vi "Swerve Wheel.vi"(7 "Wheel":T1(ring), 10 "Inputs":dbl[](array[numeric])) -> (1 "Speed":dbl, 2 "Motor Output":dbl)   [LabVIEW 2017]
uses:
  Public/Documents/Cross The Road Electronics/Phoenix-LabVIEW/Motor Controller/Controls/CTRE_Phoenix_MotorControl_ControlMode.ctl
  <vilib>/Rock Robotics/Network Tables/NT Read Number.vi
  <vilib>/Rock Robotics/Network Tables/NT Write Number.vi
  <vilib>/Rock Robotics/Network Tables/NT Read Numeric Array.vi
  <vilib>/addons/control/pid/pid.llb/PID (DBL).vi
  <vilib>/addons/control/pid/NI_PID_pid.lvlib
panel:
  out "PID Values":cluster{"P":dbl, "I":dbl, "D":dbl}
  # "Swerve Wheel Control\nFRC Team 34"
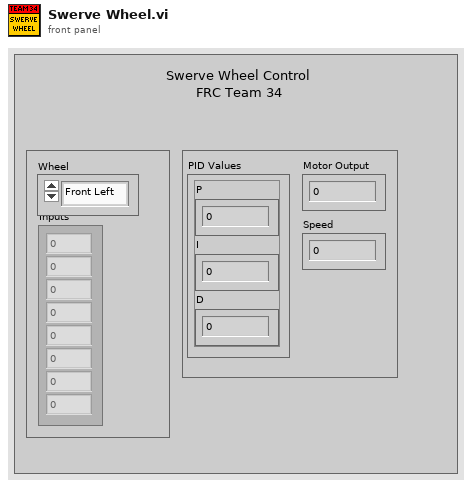
[diagram p1: front panel]
types:
  T1 = enum16{"Front Left", "Front Right", "Back Left", "Back Right"}
  T2 = typedef "CTRE_Phoenix_MotorControl_ControlMode.ctl" = u16
  T3 = enum16{"Z", "Y", "X", "Rot. Point X", "Rot. Point Y", "Width/2", "Max", "Length/2"}
  T4 = enum16{"Z Axis", "Y", "X", "Rot. Point X", "Rot. Point Y", "Width/2", "Max", "Length/2"}
  T5 = typedef "WPI_MotorControlDeviceRef.ctl" = cluster{"DeviceStatus":errorcluster, "Type":T6, "PWM":cluster{"PWM Channel":T7, "DeadBand":T8}, "CAN":cluster{"Device Number":u8, "SetOutput VI Ref":variant, "GetOutput VI Ref":variant, "Enable VI Ref":variant, "Disable VI Ref":variant, "Data":variant}, "Invert":bool, "DIO PWM":cluster{"PWM \"Enable\" Channel":T7, "DIOChannel":T9, "PWM Rate":dbl}}
  T6 = typedef "WPI_MotorControlType.ctl" = enum16{"PWM", "CAN", "DIO PWM"}
  T7 = typedef "FPGA_DIOPWMChannel.ctl" = enum8{"PWM 0", "PWM 1", "PWM 2", "PWM 3", "PWM 4", "PWM 5", "PWM 6", "PWM 7", "PWM 8", "PWM 9", "PWM MXP 0", "PWM MXP 1", "PWM MXP 2", "PWM MXP 3", "PWM MXP 4", "PWM MXP 5", "PWM MXP 6", "PWM MXP 7", "PWM MXP 8", "PWM MXP 9", "Invalid"}
  T8 = typedef "WPI_PWMDeadband.ctl" = cluster{"Name":string, "maxPositivePwm":i32, "minPositivePwm":i32, "centerPwm":i32, "maxNegativePwm":i32, "minNegativePwm":i32, "angularRange":u16}
  T9 = typedef "FPGA_DIOChannel.ctl" = enum8{"DIO 0", "DIO 1", "DIO 2", "DIO 3", "DIO 4", "DIO 5", "DIO 6", "DIO 7", "DIO 8", "DIO 9", "DIO MXP 0", "DIO MXP 1", "DIO MXP 2", "DIO MXP 3", "DIO MXP 4", "DIO MXP 5", "DIO MXP 6", "DIO MXP 7", "DIO MXP 8", "DIO MXP 9", "DIO MXP 10", "DIO MXP 11", "DIO MXP 12", "DIO MXP 13", "DIO MXP 14", "DIO MXP 15", "SPI Port CS1", "SPI Port CS2", "SPI Port CS3", "SPI Port MISO", "SPI Port MOSI", "Invalid"}
  T10 = typedef "WPI_EncoderDevRef.ctl" = cluster{"DevStatus":errorcluster, "EncoderIndex":T11, "CounterIndex":T12, "DistancePerCount":dbl, "Decoding Type":T13}
  T11 = typedef "FPGA_EncoderIdx.ctl" = enum8{"Enc 0", "Enc 1", "Enc 2", "Enc 3", "Enc 4", "Enc 5", "Enc 6", "Enc 7", "Invalid"}
  T12 = typedef "FPGA_CounterCtrSystemIndex.ctl" = enum8{"Ctr 0", "Ctr 1", "Ctr 2", "Ctr 3", "Ctr 4", "Ctr 5", "Ctr 6", "Ctr 7", "Invalid"}
  T13 = typedef "WPI_EncoderType.ctl" = enum16{"1x", "2x", "4x"}
  T14 = cluster{"Numeric":dbl, "Numeric":dbl, "Numeric":dbl}
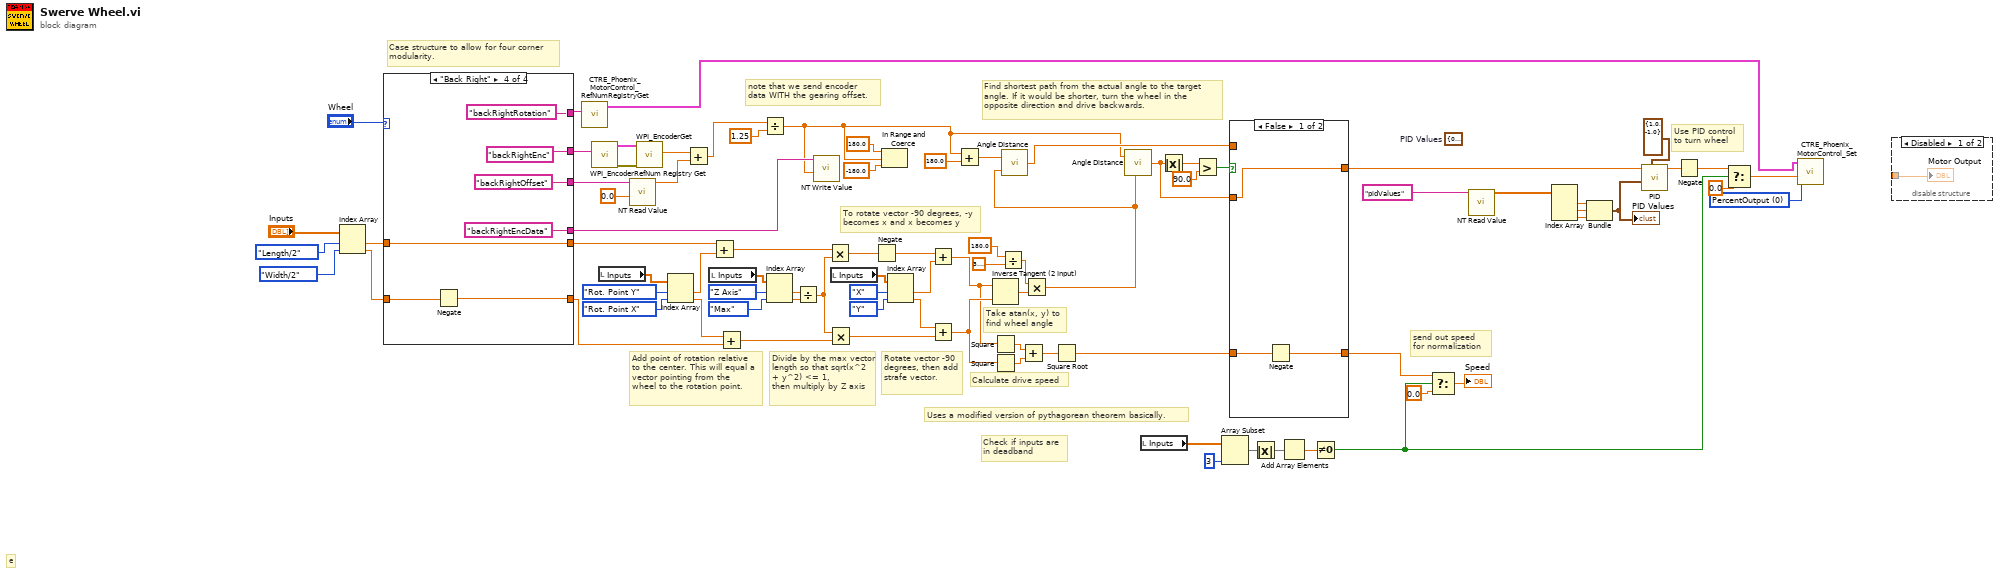
[diagram p0: block diagram]
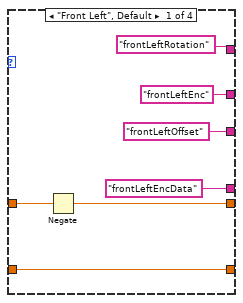
[diagram p4: hidden frame]
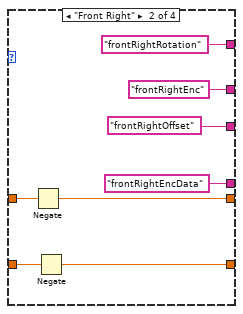
[diagram p5: hidden frame]
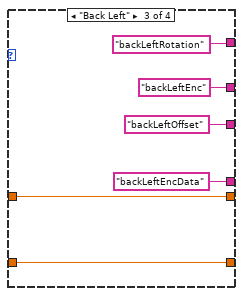
[diagram p6: hidden frame]
diagram:
  w7 = T2 0 items=["PercentOutput"=0, "Position"=1, "Velocity"=2, "Current"=3, "Follower"=5, "MotionProfile"=6, "MotionMagic"=7, "MotionMagicArc"=8, "MotionProfileArc"=10, "Disabled"=15] ("Control Mode")
  (unwired) cluster{"P":dbl, "I":dbl, "D":dbl} {"P"=0.1, "I"=0.0, "D"=0.0}  # PID Values
  # "Uses a modified version of pythagorean theorem basically."
  # "e"
  # "note that we send encoder \ndata WITH the gearing offset."
  # "Case structure to allow for four corner\nmodularity."
  # "To rotate vector -90 degrees, -y becomes x and x becomes y"
  # "send out speed\nfor normalization"
  # "Use PID control\nto turn wheel"
  # "Find shortest path from the actual angle to the target angle. If it would be shorter, turn the wheel in the opposite direction and drive backwards."
  # "Divide by the max vector length so that sqrt(x^2 + y^2) <= 1,\nthen multiply by Z axis"
  # "Add point of rotation relative to the center. This will equal a vector pointing from the\nwheel to the rotation point."
  # "Check if inputs are\nin deadband"
  # "Take atan(x, y) to find wheel angle"
  # "Calculate drive speed"
  # "Rotate vector -90 degrees, then add strafe vector."
  n1 = Index Array(array="Inputs", index #1=T3."Length/2", index #2=T3."Width/2") -> (element #1=w80:dbl, element #2=w79:dbl)
  n2 = case shown="\"Back Right\"" "Wheel" {
    tunnel: w80 -> [w91 w99 w105 w112]
    tunnel: w79 -> [w89 w97 w104 w111]
    tunnel: [w90 w98 w105 w112] -> w48
    tunnel: [w89 w96 w104 w110] -> w47
    tunnel: ["frontLeftRotation" "frontRightRotation" "backLeftRotation" "backRightRotation"] -> w10
    tunnel: ["frontLeftEnc" ("refnum name") "frontRightEnc" ("refnum name") "backLeftEnc" ("refnum name") "backRightEnc" ("refnum name")] -> w60
    tunnel: ["frontLeftOffset" ("Name") "frontRightOffset" ("Name") "backLeftOffset" ("Name") "backRightOffset" ("Name")] -> w56
    tunnel: ["frontLeftEncData" ("Name") "frontRightEncData" ("Name") "backLeftEncData" ("Name") "backRightEncData" ("Name")] -> w17
    frame "Front Left", Default {
      n3 = Negate(x=w91) -> (-x=w90:dbl)
    }
    frame "Front Right" {
      n4 = Negate(x=w99) -> (-x=w98:dbl)
      n5 = Negate(x=w97) -> (-x=w96:dbl)
    }
    frame "Back Left" {
    }
    frame "Back Right" {
      n6 = Negate(x=w111) -> (-x=w110:dbl)
    }
  }
  n7 = call "CTRE_Phoenix_MotorControl_RefNumRegistryGet.vi"("refnum name"=w10) -> ("PhoenixMotorControlDevRef"=w9:T5)  [unwired: 9 in, 1 out]
  n8 = call <vilib>:"WPI_EncoderRefNum Registry Get.vi"("refnum name"=w60) -> ("error out"=w59:errorcluster, "EncoderDevRef"=w58:T10)  [unwired: 9 in]
  n9 = local read "Inputs"() -> (w53:dbl[])
  n10 = call-poly <vilib>:"NT Read Value.vi"("Default Value"=0.0, "Name"=w56) -> ("Numeric"=w51:dbl)  [unwired: 8 in, 1 out]
  n11 = call <vilib>:"WPI_EncoderGet.vi"("error in (no error)"=w59, "EncoderDevRef"=w58) -> ("Distance"=w52:dbl)  [unwired: 4 in, 5 out]
  n12 = Index Array(array=w53, index #1=T3."Rot. Point Y", index #2=T3."Rot. Point X") -> (element #1=w49:dbl, element #2=w50:dbl)
  n13 = Add(x=w52, y=w51) -> (x+y=w16:dbl)
  n14 = local read "Inputs"() -> (w61:dbl[])
  n15 = Add(x=w48, y=w49) -> (x+y=w46:dbl)
  n16 = Add(x=w50, y=w47) -> (x+y=w71:dbl)
  n17 = Divide(x=w16, y=1.25) -> (x/y=w14:dbl)
  n18 = Index Array(array=w61, index #1=T4."Z Axis", index #2=T3."Max") -> (element #1=w19:dbl, element #2=w18:dbl)
  n19 = Divide(x=w19, y=w18) -> (x/y=w70:dbl)
  n20 = call-poly <vilib>:"NT Write Value.vi"("Numeric"=w14, "Name"=w17) -> ()  [unwired: 9 in, 1 out]
  n21 = Multiply(x=w46, y=w70) -> (x*y=w63:dbl)
  n22 = Multiply(x=w70, y=w71) -> (x*y=w66:dbl)
  n23 = local read "Inputs"() -> (w22:dbl[])
  n24 = Negate(x=w63) -> (-x=w62:dbl)
  n25 = In Range and Coerce(upper limit=180.0, x=w14, lower limit=-180.0 ("upper limit")) -> ()  [unwired: 2 out]
  n26 = Index Array(array=w22, index #1=T3."X", index #2=T3."Y") -> (element #1=w21:dbl, element #2=w20:dbl)
  n27 = Add(x=w62, y=w21) -> (x+y=w64:dbl)
  n28 = Add(x=w20, y=w66) -> (x+y=w65:dbl)
  n29 = Add(x=w14, y=180.0) -> (x+y=w43:dbl)
  n30 = Inverse Tangent (2 Input)(1:w65, 2:w64) -> (0:w78:dbl)
  n31 = Square(x=w64) -> (x^2=w67:dbl)
  n32 = Square(x=w65) -> (x^2=w77:dbl)
  n33 = Divide(x=180.0 ("y"), y=3.141592653589793) -> (x/y=w75:dbl)
  n34 = Add(x=w67, y=w77) -> (x+y=w76:dbl)
  n35 = Multiply(x=w75, y=w78) -> (x*y=w44:dbl)
  n36 = call "Angle Distance.vi"("Target Angle"=w44, "Current Angle"=w43) -> ("Distance"=w36:dbl)
  n37 = Square Root(x=w76) -> (sqrt(x)=w38:dbl)
  n38 = call "Angle Distance.vi"("Target Angle"=w44, "Current Angle"=w14) -> ("Distance"=w37:dbl)
  n39 = local read "Inputs"() -> (w32:dbl[])
  n40 = Absolute Value(x=w37) -> (abs(x)=w41:dbl)
  n41 = Greater?(x=w41, y=90.0) -> (0:w39:bool)
  n42 = Array Subset(array=w32, length=3) -> (w34:dbl[])  [unwired: 1 in]
  n43 = case shown="False" w39 {
    tunnel: w38 -> [w114 w116]
    tunnel: w37 -> [w115 _]
    tunnel: w36 -> [_ w117]
    tunnel: [w113 w116] -> w30
    tunnel: [w115 w117] -> w11
    frame False {
      n44 = Negate(x=w114) -> (-x=w113:dbl)
    }
    frame True {
    }
  }
  n45 = Absolute Value(x=w34) -> (abs(x)=w33:dbl[])
  n46 = Add Array Elements(numeric array=w33) -> (sum=w35:dbl)
  n47 = Not Equal To 0?(x=w35) -> (x != 0?=w23:bool)
  n48 = Select(t=w30, s=w23, f=0.0) -> (s? t:f=→"Speed":dbl)
  n49 = call-poly <vilib>:"NT Read Value.vi"("Name"="pidValues") -> ("Numeric Array"=w3:dbl[])  [unwired: 9 in, 1 out]
  n50 = Index Array(array=w3) -> (element #1=w6:dbl, element #2=w5:dbl, element #3=w4:dbl)  [unwired: 3 in]
  n51 = Bundle("Numeric"=w6, "Numeric"=w5, "Numeric"=w4) -> (w1:T14)  [unwired: 1 in]
  "PID Values" <- w1
  n52 = call-poly <vilib>:"PID.vi"("output range"=cluster{"output high":dbl, "output low":dbl} {"output high"=1.0, "output low"=-1.0}, "PID gains"=w1, "setpoint"=w11) -> ("output"=w26:dbl)  [unwired: 7 in, 1 out]
  n53 = Negate(x=w26) -> (-x=w24:dbl)
  n54 = Select(t=w24, s=w23, f=0.0) -> (s? t:f=w8:dbl)
  n55 = call "CTRE_Phoenix_MotorControl_Set.vi"("Output"=w8, "Control Mode"=w7, "PhoenixMotorControlDevRef"=w9) -> ()  [unwired: 7 in, 2 out]
  n56 = disable-structure shown="Disabled" {
    disable-tunnel: _ -> [w118 _]
    frame Disabled {
      "Motor Output" <- w118
    }
    frame Enabled {
    }
  }
